vi "sotring_lab_3_6.vi"() -> ()   [LabVIEW 2020]
panel:
  in  "String":string
  out "Array":string[](array[string])
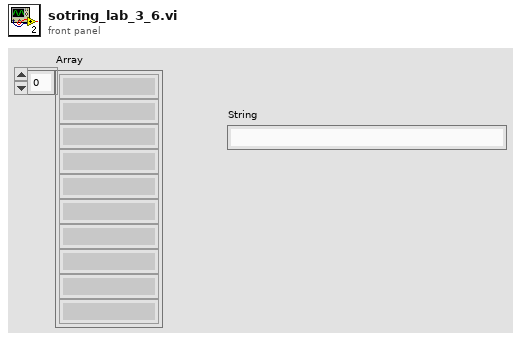
[diagram p1: front panel]
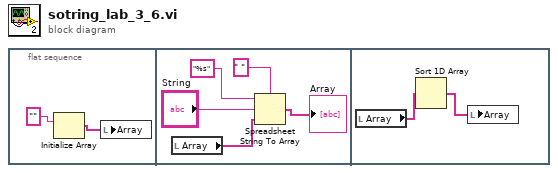
[diagram p0: block diagram]
diagram:
  n1 = flat-sequence {
    frame #0 {
      n2 = Initialize Array("") -> (w2:string[])  [unwired: 1 in]
      n3 = local write "Array"(w2) -> ()
    }
    frame #1 {
      n4 = local read "Array"() -> (w7:string[])
      n5 = Spreadsheet String To Array(delimiter (Tab)=" ", format string="%s", spreadsheet string="String", array type (2D Dbl)=w7) -> (array=→"Array":string[])
    }
    frame #2 {
      n6 = local read "Array"() -> (w8:string[])
      n7 = Sort 1D Array(array=w8) -> (sorted array=w9:string[])
      n8 = local write "Array"(w9) -> ()
    }
  }
